vi "Disconnect.vi"(6 "timeout (ms)":i32=30000, 8 "error in":errorcluster, 11 "session in":refnum<class "Session.lvclass">) -> (0 "error out":errorcluster, 2 "server errors":string, 3 "session out":refnum<class "Session.lvclass">, 5 "return code":u8)   [LabVIEW 2020, in "NI_SFTP.lvlib" / "Session.lvclass"]
doc: "Disconnects from the SFTP server."
uses:
  <vilib>/net/SFTP/Session/Session.lvclass
  <vilib>/net/SFTP/Session/Session.lvclass/Session.ctl
  <vilib>/net/SFTP/Session/Handle.ctl
  <vilib>/net/SFTP/Low Level Connection/Low Level Connection.lvclass
  <vilib>/net/SFTP/Session/Is Connected.vi
  <vilib>/net/SSH/Client/Generic/Generic Client.lvclass
  <vilib>/Utility/Deadline/NI_Deadline.lvlib
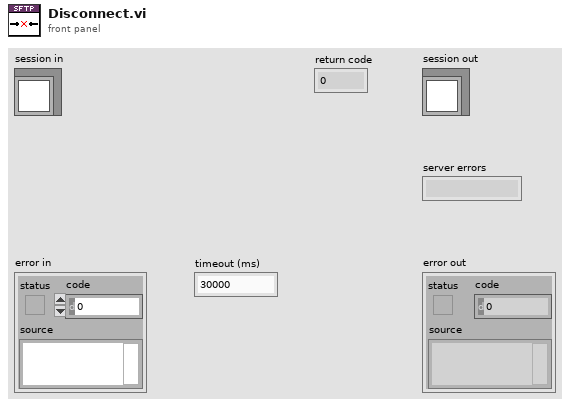
[diagram p1: front panel]
types:
  T1 = typedef "NI_Deadline.lvlib/Deadline.ctl" = cluster{"mode":T2, "deadline (ms)":u32}
  T2 = typedef "NI_Deadline.lvlib/Mode.ctl" = enum16{"Relative", "Use deadline", "Wait forever", "Nonblocking", "N/A"}
  T3 = typedef "Semaphore RefNum" = refnum<k1>
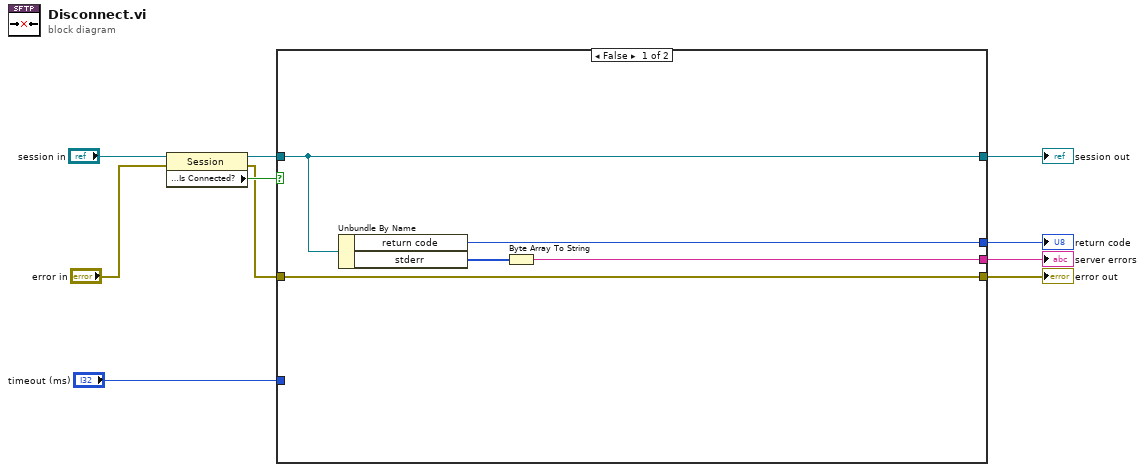
[diagram p0: block diagram]
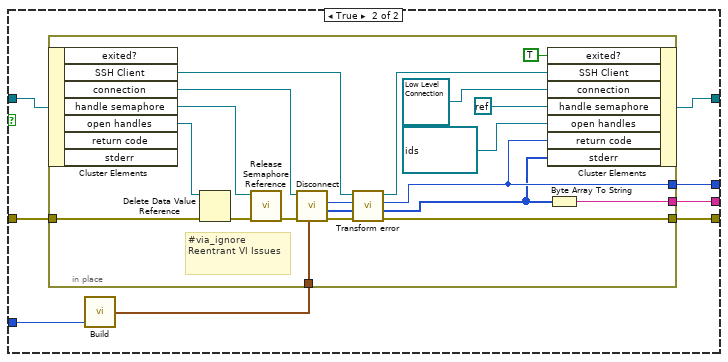
[diagram p2: hidden frame]
diagram:
  n1 = property class="Session"(reference="session in", error in="error in") -> (reference out=w4:refnum<class "Session.lvclass">, error out=w1:errorcluster, "Properties:Is Connected?"=w3:bool)
  n2 = case shown="False" w3 {
    tunnel: [w13 w23] -> w10
    tunnel: [w11 w22] -> w9
    tunnel: "timeout (ms)" -> [_ w21]
    tunnel: [w14 w19] -> w7
    tunnel: [w15 w18] -> w6
    tunnel: w1 -> [w13 w17]
    tunnel: w4 -> [w15 w16]
    frame False {
      n3 = Unbundle By Name(w15) -> ("return code"=w14:u8, "stderr"=w12:u8[])
      n4 = Byte Array To String(unsigned byte array=w12) -> (string=w11:string)
    }
    frame True {
      n5 = call <vilib>:"Build.vi"("timeout (ms)"=w21) -> ("Deadline out"=w20:T1)  [unwired: 2 in]
      n6 = in-place {
        in-place-border: [w41] -> w23
        in-place-border: [w26] -> w22
        in-place-border: w20 -> [w43]
        in-place-border: w17 -> [w31]
        in-place-border: [w27] -> w19
        # "#via_ignore Reentrant VI Issues"
        n7 = in-place-cluster #1(w16) -> ("SSH Client"=w39:refnum<class "Generic Client.lvclass">, "connection"=w37:refnum<class "Low Level Connection.lvclass">, "handle semaphore"=w35:T3, "open handles"=w34:refnum<data-value>)  [unwired: 3 out]
        n8 = Delete Data Value Reference(data value reference=w34, error in=w31) -> (error out=w30:errorcluster)  [unwired: 1 out]
        n9 = call <vilib>:"Release Semaphore Reference.vi"("error in (no error)"=w30, "semaphore"=w35) -> ("error out"=w29:errorcluster)  [unwired: 8 in, 1 out]
        n10 = call-dynamic "Disconnect.vi"("deadline"=w43, "error in"=w29, "connection in"=w37) -> ("error out"=w42:errorcluster, "server errors remaining"=w40:u8[], "return code"=w28:u8)  [unwired: 3 in, 3 out]
        n11 = call-dynamic "Transform error.vi"("error in (no error)"=w42, "server errors"=w40, "return code"=w28, "client in"=w39) -> ("error out"=w41:errorcluster, "server errors out"=w24:u8[], "return code out"=w27:u8, "client out"=w38:refnum<class "Generic Client.lvclass">)  [unwired: 4 in]
        n12 = in-place-cluster #1("exited?"=TRUE ("exit info.exited?"), "SSH Client"=w38, "connection"=refnum<class "Low Level Connection.lvclass"> refnum, "handle semaphore"=refnum<k0> refnum, "open handles"=refnum<data-value> refnum, "return code"=w27, "stderr"=w24) -> (w18:refnum<class "Session.lvclass">)
        n13 = Byte Array To String(unsigned byte array=w24) -> (string=w26:string)
      }
    }
  }
  "error out" <- w10
  "session out" <- w6
  "server errors" <- w9
  "return code" <- w7
